vi "HelpWindow.vi"   [LabVIEW 2015, in "CS++MessagemakerUtilities.lvlib"]
uses:
  CS++MessagemakerUtilities.lvlib
panel:
  # "This is the Message Maker of the CS++ framework.\n\nNote that if you want to overwrite old messages your VIs does\nnot have to be locked (because of write protection for example).\nOtherwise you will get an error message.\n\nWith this tool you can create four different types of messages:"
  # "Normal message found"
  # "Message with a CS++ Dialog"
  # "Message inherited from PVUpdate (can be send from PVs)"
  # "PVUpdate Message with Dialog option  (so option 2+3)"
  # "No information found for this message"
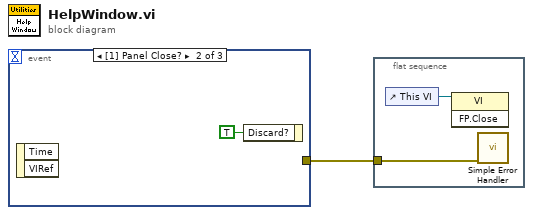
[diagram p0: block diagram]
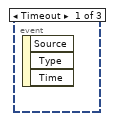
[diagram p2: hidden frame]
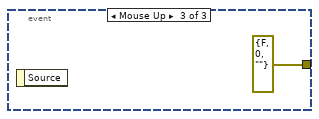
[diagram p3: hidden frame]
diagram:
  n1 = event shown="[1] Panel Close?" {
    selector: _ -> [_ _ _]
    dyn-events: _ -> [_ _ _]
    timeout: _ -> [_ _ _]
    tunnel: [_ _ errorcluster {"status"=FALSE, "code"=0, "source"=""} ("error constant")] -> w1
    event Timeout {
      n2 = event-data() -> ()  [unwired: 1 in, 3 out]
    }
    event Panel Close? {
      n3 = event-data() -> ()  [unwired: 1 in, 2 out]
      n4 = event-data("Discard?"=TRUE) -> ()  [unwired: 1 in, 1 out]
    }
    event Mouse Up {
      n5 = event-data() -> ()  [unwired: 1 in, 1 out]
    }
  }
  n6 = flat-sequence {
    tunnel: w1 -> [w5]
    frame #0 {
      n7 = control-ref of="This VI"() -> (w4:refnum<vi>)
      n8 = invoke class="VI" method="FP.Close"(reference=w4) -> ()  [unwired: 2 in, 3 out]
      n9 = call <vilib>:"Simple Error Handler.vi"("error in (no error)"=w5) -> ()  [unwired: 4 in, 5 out]
    }
  }
